vi "WriteReadMessage.vi"(0 "reference":refnum<class "VdTcpIP.lvclass">, 1 "MessageToWrite":string, 2 "timeout ms (25000)":i32=25000, 3 "Binary(F)":bool, 4 "MaxBytesToRead(10000)":i32=10000, 5 "error in (no error)":errorcluster, 7 "ReadUntilDataReceived(Ignored if not wired)":string, 9 "LockSemaphore(True)":bool=TRUE) -> (14 "reference out":refnum<class "VdTcpIP.lvclass">, 15 "ReturnedMessage":string, 17 "Reconnected":bool, 19 "error out":errorcluster)   [LabVIEW 2020, in "VdTcpIP.lvclass"]
doc: "Write and then read response\nUsing the Connect-connection"
uses:
  VdTcpIP.lvclass
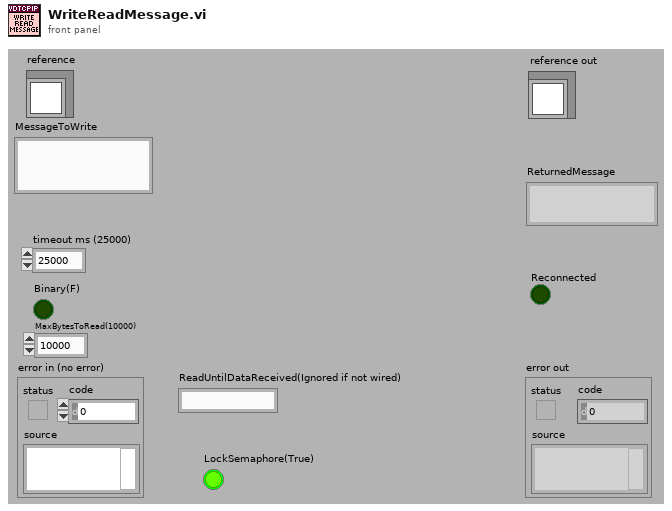
[diagram p1: front panel]
types:
  T1 = enum16{"Standard", "Buffered", "CRLF", "Immediate"}
  T2 = typedef "VdTcpIP.lvclass/ObjectAttributes.ctl" = cluster{"IP-Address":string, "Port":u16, "Connection":refnum<k5>, "Listener":refnum<k5>, "ListenerConnection":refnum<k5>, "Listner":bool, "ListnerProcessRunning":bool, "InConnections":refnum<k5>[], "InConnectionsIP":string[], "InConnectionAdded":refnum<notifier>, "RunVIOnNewConnection":variant, "DataToNewConnectionVI":cluster{"ControlName":string, "ControlValue":variant}[], "WebServicesURL_Location(http://...)":string, "WebServicesPostWebPage(*.asmx)":string, "Semaphore":T3, "AutoReConnectTimes":i32, "AutoReConnectInterval(ms)":i32, "ConnectionTimeout":i32}
  T3 = typedef "Semaphore RefNum" = refnum<k1>
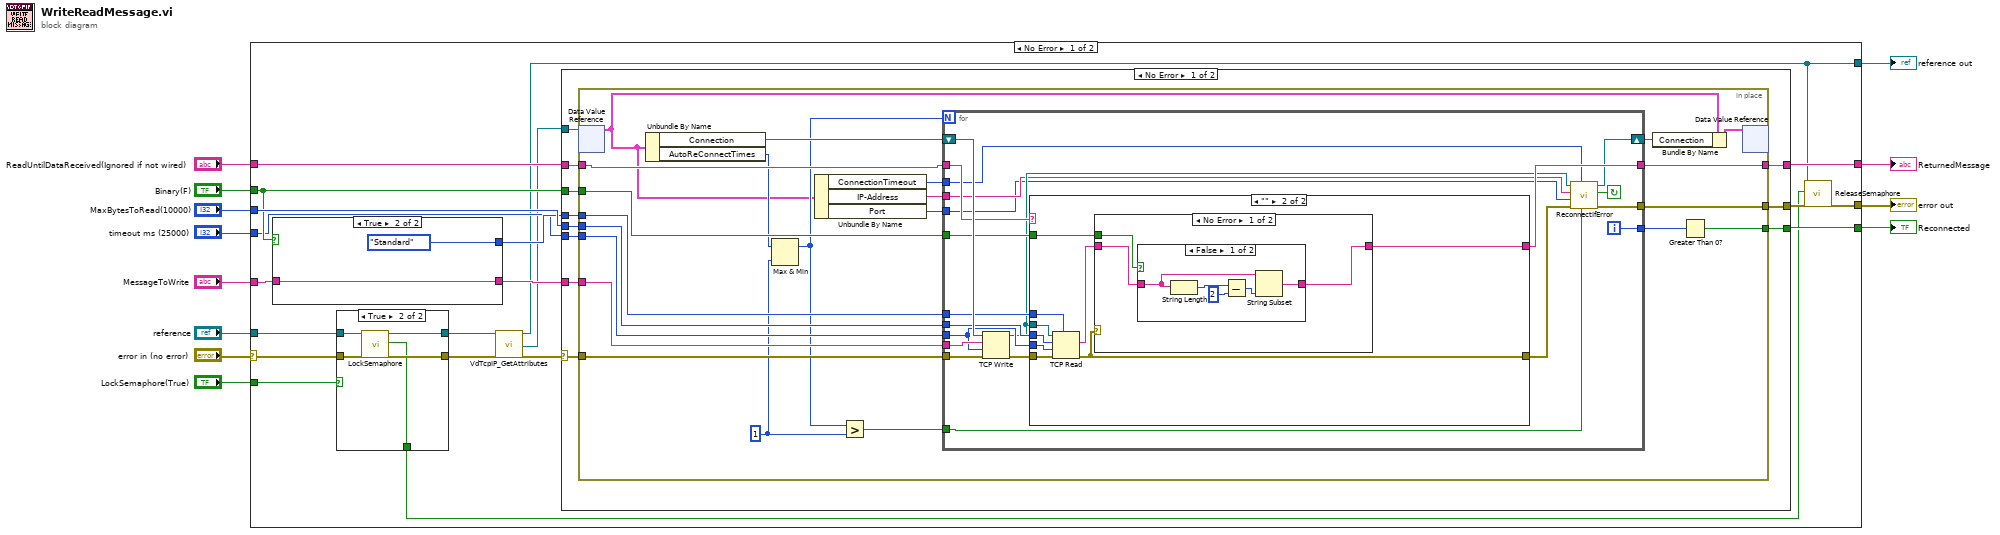
[diagram p0: block diagram]
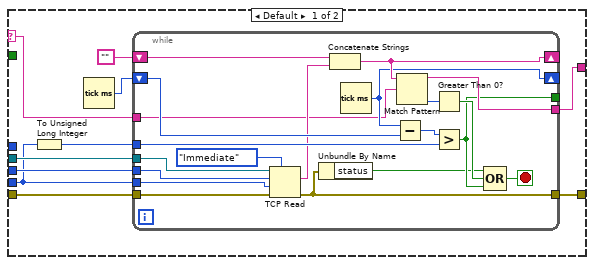
[diagram p3: hidden frame]
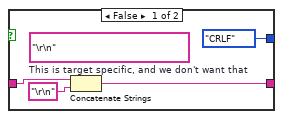
[diagram p7: hidden frame]
diagram:
  n1 = case shown="No Error" "error in (no error)" {
    selector: "error in (no error)" -> [w18 w149]
    tunnel: "reference" -> [w22 w150]
    tunnel: [w16 w149] -> w10
    tunnel: [w15 w150] -> w9
    tunnel: "MessageToWrite" -> [w31 _]
    tunnel: "timeout ms (25000)" -> [w24 _]
    tunnel: [w27 _] -> w6
    tunnel: "Binary(F)" -> [w28 _]
    tunnel: "MaxBytesToRead(10000)" -> [w29 _]
    tunnel: "ReadUntilDataReceived(Ignored if not wired)" -> [w25 _]
    tunnel: [w20 _] -> w2
    tunnel: "LockSemaphore(True)" -> [w13 _]
    frame No Error {
      n2 = case shown="True" w28 {
        tunnel: w31 -> [w146 w148]
        tunnel: [w145 w148] -> w30
        tunnel: [T1."CRLF" ("mode (standard)") T1."Standard" ("mode (standard)")] -> w26
        frame False {
          (unwired) "\r\n"  # This is target specific, and we don't want that
          n3 = Concatenate Strings(w146, "\r\n" ("string")) -> (w145:string)
        }
        frame True {
        }
      }
      n4 = case shown="True" w13 {
        tunnel: w22 -> [w34 w39]
        tunnel: [w34 w38] -> w19
        tunnel: w18 -> [w33 w37]
        tunnel: [w33 w36] -> w17
        tunnel: [_ w35] -> w14
        frame False {
        }
        frame True {
          n5 = call-dynamic "LockSemaphore.vi"("reference in"=w39, "error in (no error)"=w37) -> ("reference out"=w38:refnum<class "VdTcpIP.lvclass">, "Locked"=w35:bool, "error out"=w36:errorcluster)  [unwired: 15 in]
        }
      }
      n6 = call "VdTcpIP_GetAttributes.vi"("reference in"=w19, "error in (no error)"=w17) -> ("reference out"=w15:refnum<class "VdTcpIP.lvclass">, "DataRef"=w21:refnum<data-value>, "error out"=w32:errorcluster)  [unwired: 1 in, 14 out]
      n7 = case shown="No Error" w32 {
        selector: w32 -> [w42 w142]
        tunnel: w30 -> [w50 _]
        tunnel: w29 -> [w49 _]
        tunnel: w28 -> [w48 _]
        tunnel: [w47 _] -> w27
        tunnel: w26 -> [w46 _]
        tunnel: w25 -> [w45 _]
        tunnel: [w44 w142] -> w23
        tunnel: w24 -> [w43 _]
        tunnel: w21 -> [w41 _]
        tunnel: [w40 _] -> w20
        frame No Error {
          n8 = in-place {
            in-place-border: w50 -> [w72]
            in-place-border: w49 -> [w71]
            in-place-border: w48 -> [w70]
            in-place-border: [w69] -> w47
            in-place-border: w46 -> [w68]
            in-place-border: w45 -> [w67]
            in-place-border: [w66] -> w44
            in-place-border: w43 -> [w65]
            in-place-border: w42 -> [w64]
            in-place-border: [w60] -> w40
            w58 = 1 ("x")
            n9 = in-place-dvr #1(w41) -> (w55:T2)  [unwired: 1 out]
            n10 = Unbundle By Name(w55) -> ("Connection"=w63:refnum<k5>, "AutoReConnectTimes"=w56:i32)
            n11 = Max & Min(x=w56, y=w58) -> (max(x,y)=w59:i32)  [unwired: 1 out]
            n12 = Unbundle By Name(w55) -> ("ConnectionTimeout"=w54:i32, "IP-Address"=w53:string, "Port"=w52:u16)
            n13 = Greater?(x=w59, y=w58) -> (0:w57:bool)
            n14 = for {
              N: w59 -> [_]
              tunnel: w72 -> [w90]
              tunnel: w71 -> [w89]
              tunnel: w70 -> [w88]
              tunnel: w68 -> [w86]
              tunnel: w65 -> [w84]
              tunnel: w64 -> [w83]
              tunnel: [w75] -> w66
              shift-right: [w78] -> w62
              shift-left: w63 -> [w92]
              tunnel: w53 -> [w81]
              tunnel: w52 -> [w80]
              tunnel: w54 -> [w79]
              tunnel: [w76] -> w61
              tunnel: w57 -> [w73]
              tunnel: w67 -> [w85]
              tunnel: [w87] -> w69
              i -> [w76]
              stop <- w77 continue-if-true
              n15 = TCP Write(connection ID=w92, data in=w90, error in (no error)=w83, 9:w84) -> (connection ID out=w82:refnum<k5>, error out=w91:errorcluster)  [unwired: 1 out]
              n16 = case shown="\"\"" w85 {
                selector: w85 -> [w94 _]
                tunnel: w91 -> [w100 w131]
                tunnel: w82 -> [w99 w130]
                tunnel: w84 -> [w93 w129]
                tunnel: w89 -> [w98 w128]
                tunnel: [w97 w127] -> w74
                tunnel: w88 -> [_ w126]
                tunnel: [w96 w124] -> w87
                tunnel: w86 -> [_ w123]
                frame Default {
                  n17 = To Unsigned Long Integer(number=w93) -> (unsigned 32bit integer=w95:u32)
                  n18 = Tick Count (ms)() -> (millisecond timer value=w101:u32)
                  n19 = while {
                    tunnel: w98 -> [w111]
                    tunnel: w95 -> [w114]
                    tunnel: [w112] -> _
                    tunnel: [w106] -> w97
                    tunnel: w100 -> [w115]
                    shift-left: w101 -> [w116]
                    shift-right: [w108] -> _
                    tunnel: [w120] -> w96
                    shift-left: "" -> [w117]
                    shift-right: [w109] -> _
                    tunnel: w99 -> [w122]
                    tunnel: w94 -> [w104]
                    tunnel: w93 -> [w103]
                    stop <- w107 stop-if-true
                    n20 = TCP Read(connection ID=w122, bytes to read=w111, error in (no error)=w115, 7:T1."Immediate" ("mode (standard)"), 9:w103) -> (data out=w110:string, error out=w106:errorcluster)  [unwired: 1 out]
                    n21 = Unbundle By Name(w106) -> ("status"=w105:bool)
                    n22 = Concatenate Strings(w117, w110) -> (w109:string)
                    n23 = Tick Count (ms)() -> (millisecond timer value=w108:u32)
                    n24 = Subtract(x=w108, y=w116) -> (x-y=w119:u32)
                    n25 = Match Pattern(string=w109, regular expression=w104) -> (before substring=w120:string, offset past match=w121:i32)  [unwired: 3 out]
                    n26 = Greater Than 0?(x=w121) -> (x > 0?=w118:bool)
                    n27 = Greater?(x=w119, y=w114) -> (0:w112:bool)
                    n28 = Compound Arithmetic op=OR(w105, w118, w112) -> (w107:bool)
                  }
                }
                frame "" {
                  n29 = TCP Read(connection ID=w130, bytes to read=w128, error in (no error)=w131, 7:w123, 9:w129) -> (data out=w125:string, error out=w127:errorcluster)  [unwired: 1 out]
                  n30 = case shown="No Error" w127 {
                    tunnel: w125 -> [w133 w141]
                    tunnel: w126 -> [w134 _]
                    tunnel: [w132 w141] -> w124
                    frame No Error {
                      n31 = case shown="False" w134 {
                        tunnel: w133 -> [w139 w140]
                        tunnel: [w135 w140] -> w132
                        frame False {
                          n32 = String Length(string=w139) -> (length=w138:i32)
                          n33 = Subtract(x=w138, y=2) -> (x-y=w136:i32)
                          n34 = String Subset(string=w139, length (rest)=w136) -> (substring=w135:string)  [unwired: 1 out]
                        }
                        frame True {
                        }
                      }
                    }
                    frame Error {
                    }
                  }
                }
              }
              n35 = call "ReconnectIfError.vi"("TryReconnect"=w73, "ConnectionTimeout"=w79, "error in (no error)"=w74, "Port"=w80, "IP-Address"=w81, "TCP Network Connection in"=w82) -> ("error out"=w75:errorcluster, "TryAgain(Managed to Reconnect, and TryReconnect is True)"=w77:bool, "TCP Network Connection out"=w78:refnum<k5>)  [unwired: 3 in]
            }
            n36 = Bundle By Name(cluster=w55, "Connection"=w62) -> (w51:T2)
            n37 = Greater Than 0?(x=w61) -> (x > 0?=w60:bool)
            n38 = in-place-dvr #1(w51) -> ()  [unwired: 2 out]
          }
        }
        frame Error {
        }
      }
      n39 = call-dynamic "ReleaseSemaphore.vi"("reference in"=w15, "ManagedToLockIt"=w14, "error in (no error)"=w23) -> ("error out"=w16:errorcluster)  [unwired: 15 in, 1 out]
    }
    frame Error {
    }
  }
  "reference out" <- w9
  "error out" <- w10
  "ReturnedMessage" <- w6
  "Reconnected" <- w2
